vi "Acquire Instrument.vi"(8 "error in (no error)":errorcluster caption="entrée d'erreur (pas d'erreur)", 11 "Class Instrument (Default) en entrée":refnum<class "Class Instrument (Default).lvclass">) -> (0 "error out":errorcluster caption="sortie d'erreur", 3 "Class Instrument (Default) en sortie":refnum<class "Class Instrument (Default).lvclass">)   [LabVIEW 2020, in "Library Instrument & Equipement.lvlib" / "Library Instruments.lvlib" / "Class Instrument (Default).lvclass"]
doc: "Action to be taken after each series of actions (Autotest, Read, Write, ...)\nNo need to use this action before the close instrument function"
uses:
  Class Instrument (Default).lvclass
  Commun VI/TypeDef/Liste Error.ctl
  Commun VI/Library Commun.lvlib
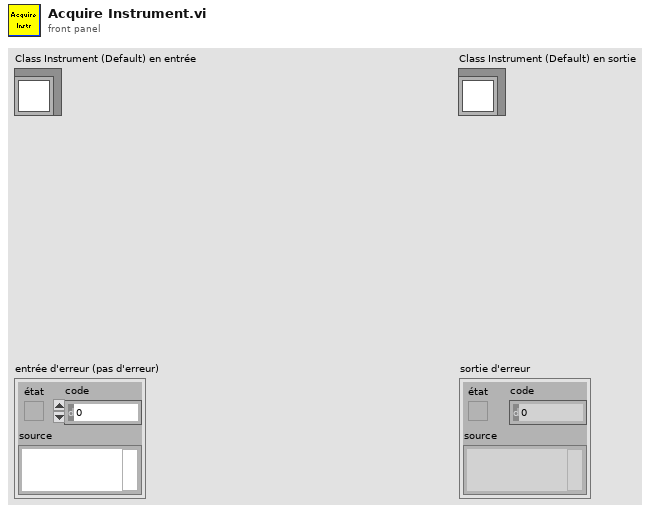
[diagram p1: front panel]
types:
  T1 = typedef "Library Commun.lvlib/Liste Error.ctl" = enum16{"Firebase Driver - Get Document", "Firebase Driver - Get Document With Where", "Firebase Driver - Delete Document", "Firebase Driver - Set Document", "Firebase Driver - Update Document", "Firebase Altyor - Search Document Bench", "Firebase Altyor - Class Not in Firebase", "Spectrum_Analyser - Timeout", "Relay Board - Qty Relay", "DIO - Pb Funtion", "Power_Supply - Peripherical not find", "Mutimeter - Peripherical not find", "Instrument - Function Not Used", "Instrument - Instrument name not specified", "Instrument - Allready Initialised", "Instrument - TimeOut", "Instrument - the instrument must be Initialise before", "Instrument - Frame Not received", "Instrument - Frame Nok", "Test - Initialise the File_for_Save", "Test - Timeout", "Test - Cmd Error", "FGV - Variable ", "BDD FireBase - Define Class", "SN - Class Not Define"}
  T2 = typedef "Semaphore RefNum" = refnum<k1>
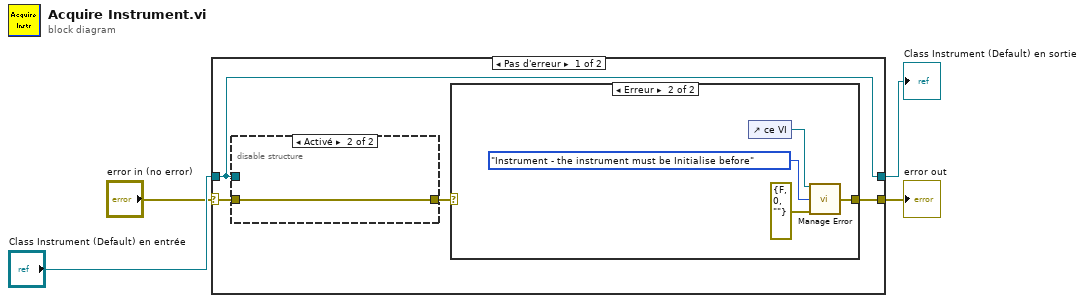
[diagram p0: block diagram]
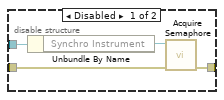
[diagram p2: hidden frame]
diagram:
  n1 = case shown="Pas d'erreur" "error in (no error)" {
    selector: "error in (no error)" -> [w7 w20]
    tunnel: [w6 w20] -> w2
    tunnel: [w8 w19] -> w1
    tunnel: "Class Instrument (Default) en entrée" -> [w8 w19]
    frame No Error {
      n2 = disable-structure shown="Activé" {
        disable-tunnel: w8 -> [w12 _]
        disable-tunnel: w7 -> [w11 w13]
        disable-tunnel: [w10 w13] -> w5
        frame Disabled {
          n3 = Unbundle By Name(w12) -> ("Synchro Instrument"=w9:T2)
          n4 = call <vilib>:"Acquire Semaphore.vi"("error in (no error)"=w11, "semaphore"=w9) -> ("error out"=w10:errorcluster)  [unwired: 3 in, 2 out]
        }
        frame Enabled {
        }
      }
      n5 = case shown="Erreur" w5 {
        selector: w5 -> [w14 _]
        tunnel: [w14 w16] -> w6
        frame No Error {
        }
        frame Error {
          n6 = control-ref of="ce VI"() -> (w18:refnum<vi>)
          n7 = call "Manage Error.vi"("VI in Error"=w18, "Code Erreur"=Liste_Error."Instrument - the instrument must be Initialise before", "error in (no error)"=errorcluster {"status"=FALSE, "code"=0, "source"=""}) -> ("error out"=w16:errorcluster)  [unwired: 12 in]
        }
      }
    }
    frame Error {
    }
  }
  "error out" <- w2
  "Class Instrument (Default) en sortie" <- w1
